vi "Write Start  Stop Actions.vi"(9 "Stop Action":T1, 10 "Start Action":T1, 11 "Valve in":refnum<class "Valve.lvclass">) -> (3 "Valve out":refnum<class "Valve.lvclass">)   [LabVIEW 2015, in "cRIO-Carbondioxide.lvlib" / "CO2-Actor.lvlib" / "Valve.lvclass"]
uses:
  Valve.lvclass
  Action.ctl
  Valve.lvclass/Valve.ctl
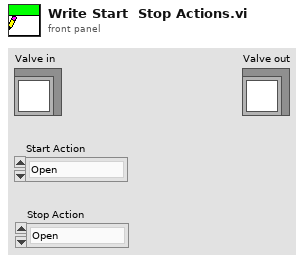
[diagram p1: front panel]
types:
  T1 = typedef "Action.ctl" = enum16{"Open", "Close", "None"}
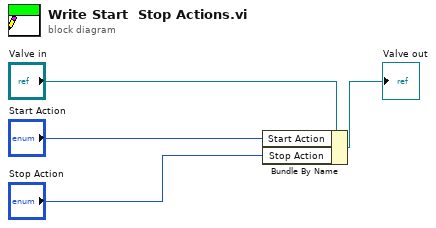
[diagram p0: block diagram]
diagram:
  n1 = Bundle By Name(cluster="Valve in", "Start Action"="Start Action", "Stop Action"="Stop Action") -> (→"Valve out":refnum<class "Valve.lvclass">)
